vi "Read File.vi"(8 "error in (no error)":errorcluster, 10 "Parameters":refnum<class "Parameter.lvclass">[](array[class]), 11 "Parameter INI File in":refnum<class "Parameter INI File.lvclass">) -> (0 "error out":errorcluster, 2 "Parameters":refnum<class "Parameter.lvclass">[](array[class]), 3 "Parameter INI File out":refnum<class "Parameter INI File.lvclass">)   [LabVIEW 2019, in "CD Parameter Manager API.lvlib" / "Parameter INI File.lvclass"]
uses:
  Parameter INI File.lvclass
  Parameter Class/Parameter.lvclass
  Parameter INI File.lvclass/Parameter INI File.ctl
  Double Parameter Class/Double Parameter.lvclass
  C:/Repositories/UI-Control-Initializer-API/Source/Parameter Class/Parameter.lvclass
  Parameter Class/Parameter.lvclass/Parameter.ctl
  Double Parameter Class/Double Parameter.lvclass/Double Parameter.ctl
  Boolean Parameter Class/Boolean Parameter.lvclass
  Boolean Parameter Class/Boolean Parameter.lvclass/Boolean Parameter.ctl
  I32 Parameter Class/I32 Parameter.lvclass
  I32 Parameter Class/I32 Parameter.lvclass/I32 Parameter.ctl
  Parameter Class/Member Accessors/Read Control label.vi
  Double Parameter Class/Member Accessors/Read Value.vi
  Parameter Class/Member Accessors/Write Control label.vi
  Double Parameter Class/Member Accessors/Write Value.vi
  Boolean Parameter Class/Member Accessors/Read Value.vi
  Boolean Parameter Class/Member Accessors/Write Value.vi
  I32 Parameter Class/Member Accessors/Read Value.vi
  I32 Parameter Class/Member Accessors/Write Value.vi
  <vilib>/Utility/config.llb/Read Key (Double).vi
  <vilib>/Utility/config.llb/Read Key (Boolean).vi
  <vilib>/Utility/config.llb/Read Key (I32).vi
  <vilib>/Utility/error.llb/Error Cluster From Error Code.vi
  <vilib>/ErrorRing/Error Ring.xnode
  <vilib>/Utility/config.llb/NI_LVConfig.lvlib
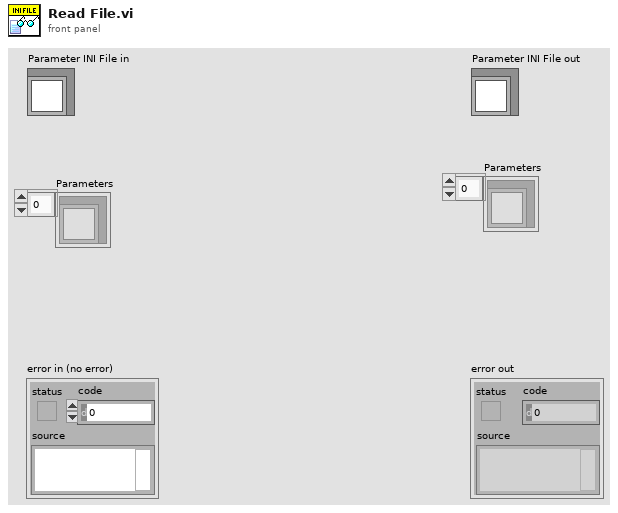
[diagram p1: front panel]
types:
  T1 = typedef "NI_LVConfig.lvlib/Config Data RefNum.ctl" = refnum<k1>
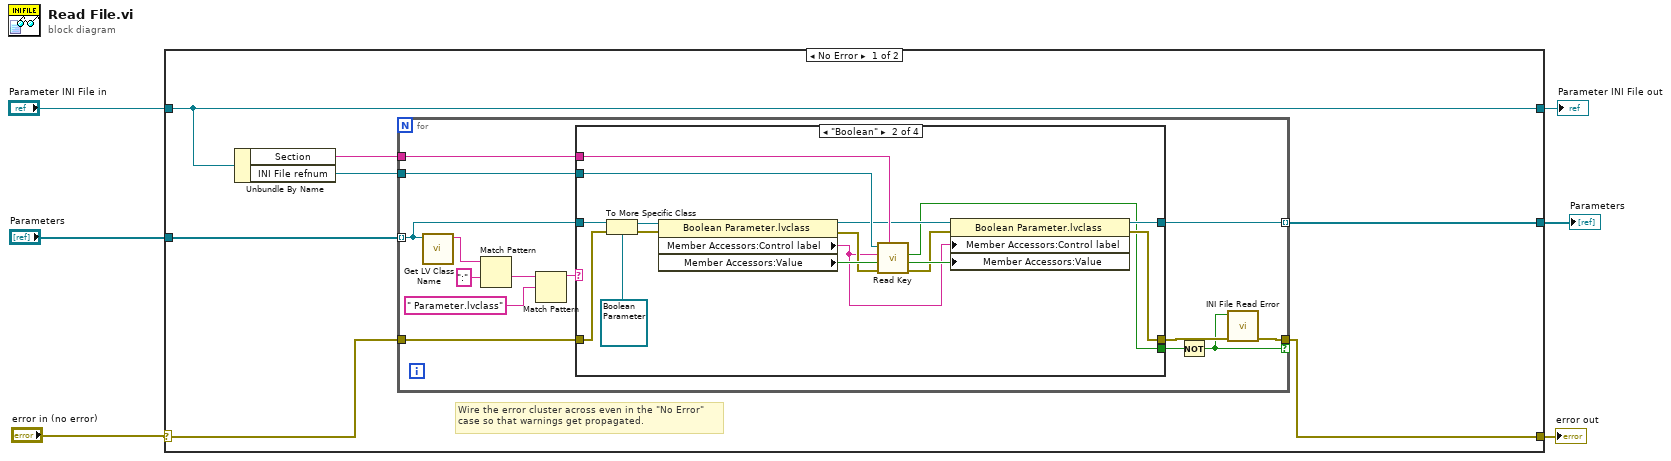
[diagram p0: block diagram]
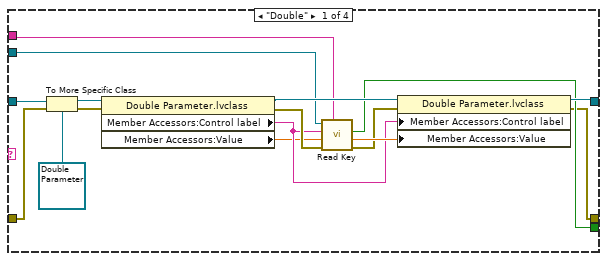
[diagram p2: hidden frame]
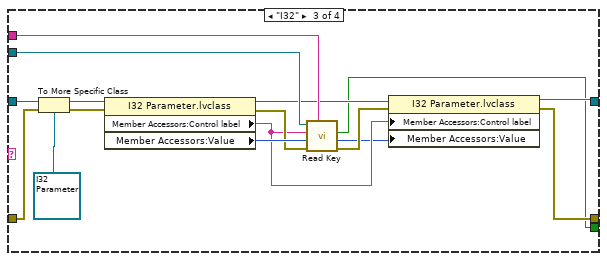
[diagram p3: hidden frame]
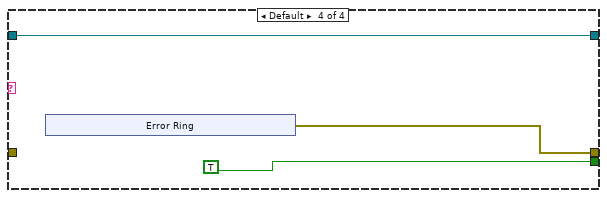
[diagram p4: hidden frame]
diagram:
  n1 = case shown="No Error" "error in (no error)" {
    selector: "error in (no error)" -> [w13 w86]
    tunnel: [w8 w86] -> w4
    tunnel: [w10 w85] -> w5
    tunnel: "Parameter INI File in" -> [w10 w85]
    tunnel: "Parameters" -> [w9 w84]
    tunnel: [w7 w84] -> w1
    frame No Error {
      # "Wire the error cluster across even in the \"No Error\"\ncase so that warnings get propagated."
      n2 = Unbundle By Name(w10) -> ("Section"=w11:string, "INI File refnum"=w12:T1)
      n3 = for {
        tunnel: w13 -> [w22]
        tunnel: [w15] -> w8 if=w14
        tunnel: w12 -> [w20]
        tunnel: w9 -> [w19] mode=indexing
        tunnel: w11 -> [w18]
        tunnel: [w17] -> w7 mode=indexing
        n4 = call <vilib>:"Get LV Class Name.vi"("object"=w19) -> ("class name"=w24:string)  [unwired: 9 in, 1 out]
        n5 = Match Pattern(string=w24, regular expression=":") -> (after substring=w26:string)  [unwired: 1 in, 3 out]
        n6 = Match Pattern(string=w26, regular expression=" Parameter.lvclass") -> (before substring=w23:string)  [unwired: 1 in, 3 out]
        n7 = case shown="\"Boolean\"" w23 {
          tunnel: w22 -> [w39 w55 w71 _]
          tunnel: [w30 w46 w62 w77] -> w16
          tunnel: [w31 w44 w60 TRUE] -> w21
          tunnel: w20 -> [w28 w52 w69 _]
          tunnel: w19 -> [w42 w56 w72 w76]
          tunnel: w18 -> [w29 w53 w68 _]
          tunnel: [w32 w45 w65 w76] -> w17
          frame "Double" {
            n8 = To More Specific Class(target class=refnum<class "Double Parameter.lvclass"> refnum ("CD Parameter Manager API.lvlib:Double Parameter.lvclass"), reference=w42, error in=w39) -> (specific class reference=w41:refnum<class "Double Parameter.lvclass">, error out=w43:errorcluster)
            n9 = property class="Double Parameter.lvclass"(reference=w41, error in=w43) -> (reference out=w36:refnum<class "Double Parameter.lvclass">, error out=w35:errorcluster, "Member Accessors:Control label"=w34:string, "Member Accessors:Value"=w33:dbl)
            n10 = call-poly <vilib>:"Read Key.vi"("section"=w29, "error in (no error)"=w35, "default value"=w33, "key"=w34, "refnum"=w28) -> ("error out"=w37:errorcluster, "value"=w38:dbl, "found?"=w31:bool)  [unwired: 3 in, 1 out]
            n11 = property class="Double Parameter.lvclass"(reference=w36, error in=w37, "Member Accessors:Control label"=w34, "Member Accessors:Value"=w38) -> (reference out=w32:refnum<class "Double Parameter.lvclass">, error out=w30:errorcluster)
          }
          frame "Boolean" {
            n12 = To More Specific Class(target class=refnum<class "Boolean Parameter.lvclass"> refnum ("CD Parameter Manager API.lvlib:Boolean Parameter.lvclass"), reference=w56, error in=w55) -> (specific class reference=w58:refnum<class "Boolean Parameter.lvclass">, error out=w59:errorcluster)
            n13 = property class="Boolean Parameter.lvclass"(reference=w58, error in=w59) -> (reference out=w48:refnum<class "Boolean Parameter.lvclass">, error out=w54:errorcluster, "Member Accessors:Control label"=w47:string, "Member Accessors:Value"=w57:bool)
            n14 = call-poly <vilib>:"Read Key.vi"("section"=w53, "error in (no error)"=w54, "default value"=w57, "key"=w47, "refnum"=w52) -> ("error out"=w49:errorcluster, "value"=w50:bool, "found?"=w44:bool)  [unwired: 3 in, 1 out]
            n15 = property class="Boolean Parameter.lvclass"(reference=w48, error in=w49, "Member Accessors:Control label"=w47, "Member Accessors:Value"=w50) -> (reference out=w45:refnum<class "Boolean Parameter.lvclass">, error out=w46:errorcluster)
          }
          frame "I32" {
            n16 = To More Specific Class(target class=refnum<class "I32 Parameter.lvclass"> refnum ("CD Parameter Manager API.lvlib:I32 Parameter.lvclass"), reference=w72, error in=w71) -> (specific class reference=w74:refnum<class "I32 Parameter.lvclass">, error out=w75:errorcluster)
            n17 = property class="I32 Parameter.lvclass"(reference=w74, error in=w75) -> (reference out=w66:refnum<class "I32 Parameter.lvclass">, error out=w70:errorcluster, "Member Accessors:Control label"=w63:string, "Member Accessors:Value"=w73:i32)
            n18 = call-poly <vilib>:"Read Key.vi"("section"=w68, "error in (no error)"=w70, "default value"=w73, "key"=w63, "refnum"=w69) -> ("error out"=w64:errorcluster, "value"=w61:i32, "found?"=w60:bool)  [unwired: 3 in, 1 out]
            n19 = property class="I32 Parameter.lvclass"(reference=w66, error in=w64, "Member Accessors:Control label"=w63, "Member Accessors:Value"=w61) -> (reference out=w65:refnum<class "I32 Parameter.lvclass">, error out=w62:errorcluster)
          }
          frame Default {
            n20 = xnode "Error Ring"() -> ("error out"=w77:errorcluster)
          }
        }
        n21 = Not(x=w21) -> (.not. x?=w14:bool)
        n22 = call "INI File Read Error.vi"("error in (no error)"=w16, "INI Key Not Found?"=w14) -> ("error out"=w15:errorcluster)  [unwired: 9 in]
      }
    }
    frame Error {
    }
  }
  "error out" <- w4
  "Parameter INI File out" <- w5
  "Parameters" <- w1
